vi "Execution.vi"() -> ()   [LabVIEW 2014]
panel:
  in  "x":dbl
  out "ciclos":dbl
  in  "stop":bool
  in  "Led sequence":bool
  out "Led3":bool
  out "Led2":bool
  out "Led1":bool
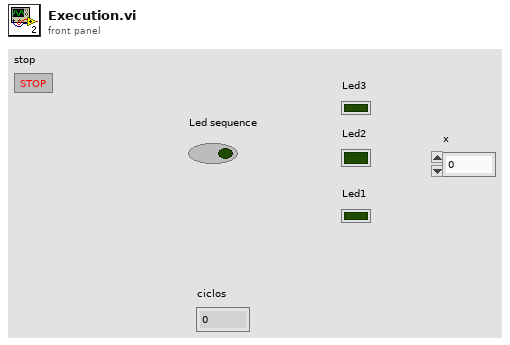
[diagram p1: front panel]
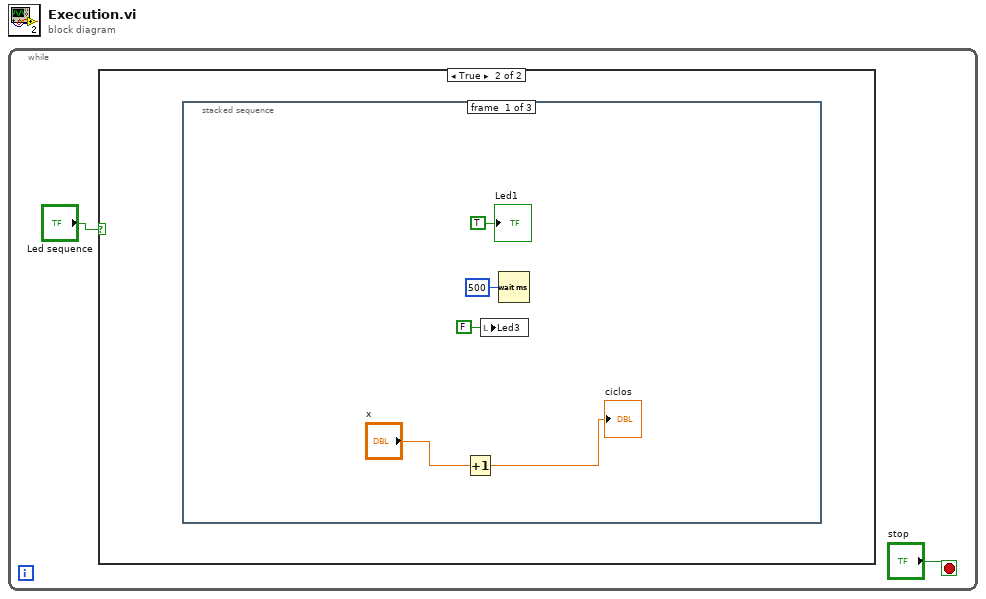
[diagram p0: block diagram]
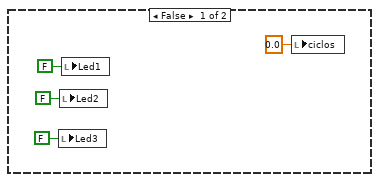
[diagram p2: hidden frame]
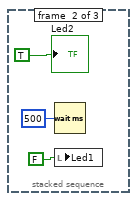
[diagram p3: hidden frame]
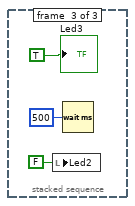
[diagram p4: hidden frame]
diagram:
  n1 = while {
    stop <- "stop" stop-if-true
    n2 = case shown="True" "Led sequence" {
      frame False {
        n3 = local write "Led3"(FALSE ("Led3")) -> ()
        n4 = local write "Led2"(FALSE ("Led2")) -> ()
        n5 = local write "Led1"(FALSE ("Led1")) -> ()
        n6 = local write "ciclos"(0.0 ("ciclos")) -> ()
      }
      frame True {
        n7 = stacked-sequence {
          frame #0 {
            n8 = Increment(x="x") -> (x+1=→"ciclos":dbl)
            n9 = local write "Led3"(FALSE ("Led3")) -> ()
            n10 = Wait (ms)(milliseconds to wait=u32 500) -> ()  [unwired: 1 out]
            "Led1" <- TRUE ("Led1")
          }
          frame #1 {
            n11 = Wait (ms)(milliseconds to wait=u32 500) -> ()  [unwired: 1 out]
            n12 = local write "Led1"(FALSE ("Led1")) -> ()
            "Led2" <- TRUE ("Led2")
          }
          frame #2 {
            n13 = local write "Led2"(FALSE ("Led2")) -> ()
            n14 = Wait (ms)(milliseconds to wait=u32 500) -> ()  [unwired: 1 out]
            "Led3" <- TRUE ("Led3")
          }
        }
      }
    }
  }
